vi "Set_timestamp.vi"(6 "Eingang 5":dbl, 8 "Eingang 4":dbl, 9 "Eingang 3":dbl, 10 "Eingang 2":dbl, 11 "Eingang":dbl) -> (0 "Ausgang 4":waveform(dbl), 1 "Ausgang 3":waveform(dbl), 2 "Ausgang 2":waveform(dbl), 3 "Ausgang":waveform(dbl), 4 "Ausgang 5":waveform(dbl))   [LabVIEW 2015]
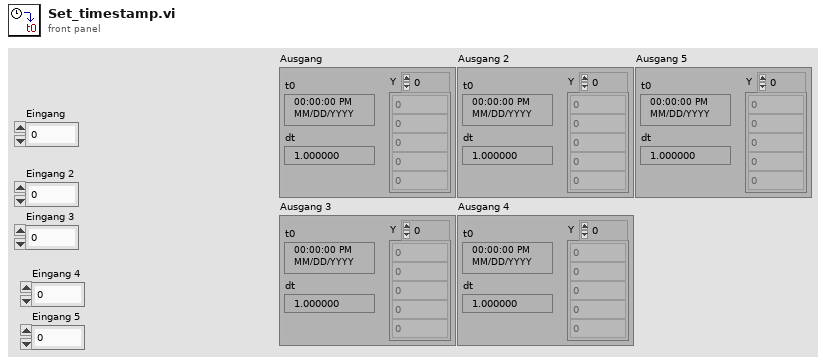
[diagram p1: front panel]
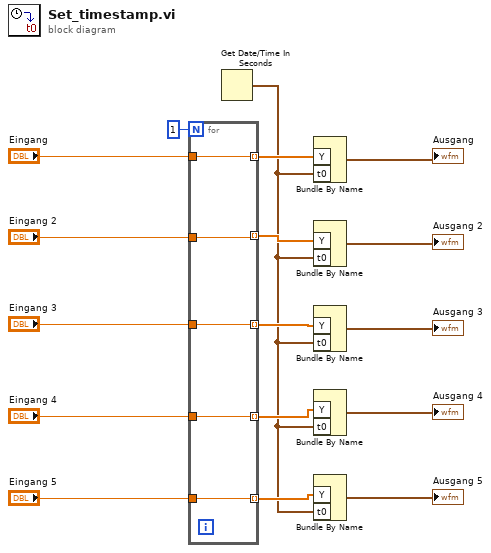
[diagram p0: block diagram]
diagram:
  n1 = for {
    N: 1 -> [_]
    tunnel: "Eingang" -> [w22]
    tunnel: [w22] -> w15 mode=indexing
    tunnel: [w21] -> w12 mode=indexing
    tunnel: "Eingang 2" -> [w21]
    tunnel: [w20] -> w11 mode=indexing
    tunnel: "Eingang 3" -> [w20]
    tunnel: [w19] -> w9 mode=indexing
    tunnel: "Eingang 4" -> [w19]
    tunnel: [w18] -> w7 mode=indexing
    tunnel: "Eingang 5" -> [w18]
  }
  n2 = Get Date/Time In Seconds() -> (seconds since 1Jan1904=w5:timestamp)
  n3 = Bundle By Name("Y"=w15, "t0"=w5) -> (→"Ausgang":waveform(dbl))  [unwired: 1 in]
  n4 = Bundle By Name("Y"=w12, "t0"=w5) -> (→"Ausgang 2":waveform(dbl))  [unwired: 1 in]
  n5 = Bundle By Name("Y"=w11, "t0"=w5) -> (→"Ausgang 3":waveform(dbl))  [unwired: 1 in]
  n6 = Bundle By Name("Y"=w9, "t0"=w5) -> (→"Ausgang 4":waveform(dbl))  [unwired: 1 in]
  n7 = Bundle By Name("Y"=w7, "t0"=w5) -> (→"Ausgang 5":waveform(dbl))  [unwired: 1 in]
